vi "Format_into_string.vi"() -> ()   [LabVIEW 2019]
panel:
  in  "Tamil Nadu":u32=5198
  in  "Month":string="May"
  in  "Gujrat":u32=5234
  in  "Mahararstra":u32=15649
  out "Output string":string
  in  "Year":u32=2020
  in  "Day":u32=10
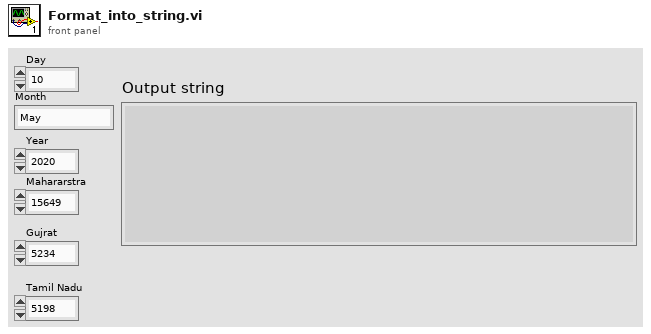
[diagram p1: front panel]
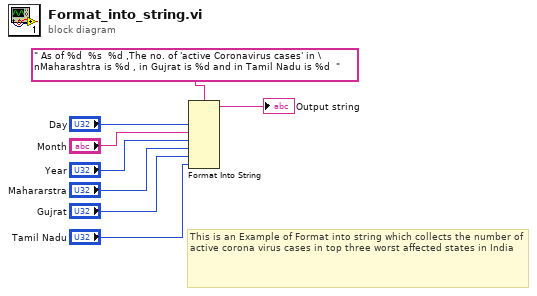
[diagram p0: block diagram]
diagram:
  # "This is an Example of Format into string which collects the number of active corona virus cases in top three worst affected states in India"
  n1 = Format Into String(format string=" As of %d  %s  %d ,The no. of 'active Coronavirus cases' in \nMaharashtra is %d , in Gujrat is %d and in Tamil Nadu is %d  ", "Day", "Month", "Year", "Mahararstra", "Gujrat", "Tamil Nadu") -> (resulting string=→"Output string":string)  [unwired: 2 in, 1 out]
